vi "VI-Create XControl State Controls.vi"(0 "Path":path=path "C:/Users/hancock/Desktop/Test/Test.xctl", 11 "error in (no error)":errorcluster) -> (6 "Names":string[](array[string]), 8 "Data Types":variant[](array[variant]), 15 "error out":errorcluster)   [LabVIEW 2015]
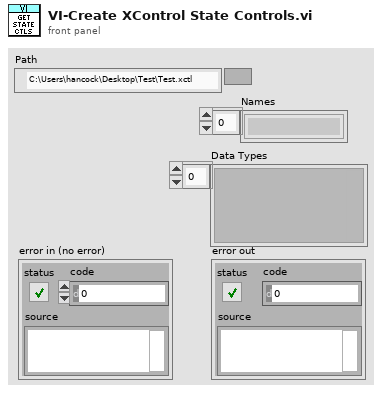
[diagram p1: front panel]
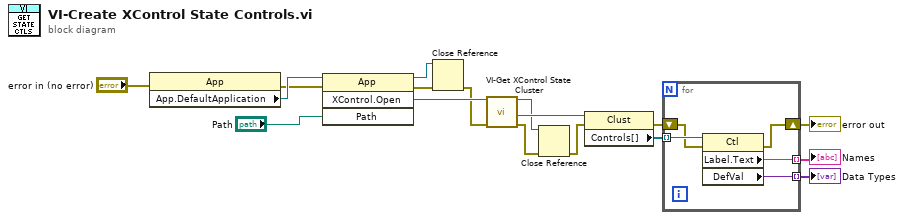
[diagram p0: block diagram]
diagram:
  n1 = property class="App"(error in="error in (no error)") -> (error out=w13:errorcluster, "App.DefaultApplication"=w14:refnum<vi>)  [unwired: 1 in, 1 out]
  n2 = invoke class="App" method="XControl.Open"(reference=w14, error in=w13, "Path"="Path") -> (reference out=w6:refnum<vi>, error out=w7:errorcluster, "Open XControl"=w16:refnum<vi>)  [unwired: 1 in, 1 out]
  n3 = Close Reference(reference=w6, error in (no error)=w7) -> (error out=w5:errorcluster)
  n4 = call "VI-Get XControl State Cluster.vi"("XControlLibrary in"=w16, "error in (no error)"=w5) -> ("XControlLibrary out"=w1:refnum<vi>, "State cluster"=w4:refnum<vi>, "error out"=w3:errorcluster)  [unwired: 10 in, 1 out]
  n5 = Close Reference(reference=w1, error in (no error)=w3) -> (error out=w2:errorcluster)
  n6 = property class="Clust"(reference=w4, error in=w2) -> (error out=w10:errorcluster, "Controls[]"=w12:refnum<vi>[])  [unwired: 1 out]
  n7 = for {
    tunnel: w12 -> [w22] mode=indexing
    tunnel: [w21] -> w11 mode=indexing
    shift-right: [w19] -> w9
    shift-left: w10 -> [w20]
    tunnel: [w18] -> w8 mode=indexing
    n8 = property class="Ctl"(reference=w22, error in=w20) -> (error out=w19:errorcluster, "Label.Text"=w21:string, "DefVal"=w18:variant)  [unwired: 1 out]
  }
  "error out" <- w9
  "Names" <- w11
  "Data Types" <- w8
